vi "chem_shift.vi"() -> ()   [LabVIEW 2014]
uses:
  <vilib>/Analysis/6fits.llb/Curve Fitting Criteria.ctl
  <vilib>/Utility/file.llb/Write To Spreadsheet File (I64).vi
  <vilib>/Utility/file.llb/Write To Spreadsheet File (DBL).vi
  <vilib>/Analysis/NI_AALPro.lvlib
panel:
  in  "semester":string(combo)="ws17"
  out "ppm4":dbl=nan format="%.1f"
  out "peak4 [Hz]":dbl=nan format="%.1f"
  in  "W4-high [Hz]":i32
  in  "W4-low [Hz]":i32
  out "ppm3":dbl=nan format="%.1f"
  out "peak3 [Hz]":dbl=nan format="%.1f"
  in  "W3-high [Hz]":i32
  in  "W3-low [Hz]":i32
  out "ppm2":dbl=nan format="%.1f"
  out "peak2 [Hz]":dbl=nan format="%.1f"
  in  "W2-high [Hz]":i32
  in  "W2-low [Hz]":i32
  out "XY Graph":cluster{"Y":dbl[], "Y":dbl[]}[](graph)
  in  "meas":bool=TRUE
  out "Amplitude":cluster{"Y":dbl[], "Y":dbl[]}[](graph)
  out "Fourier transform":cluster{"Y":dbl[], "Y":dbl[]}[](graph)
  out "ppm1":dbl=nan format="%.1f"
  out "peak1 [Hz]":dbl=nan format="%.1f"
  out "offset":i32=4
  out "del freq":u32=2
  in  "W1-high [Hz]":i32
  in  "W1-low [Hz]":i32
  in  "fit:":bool=TRUE
  in  "folder":string
  in  "data file":string
  in  "scan freq [kHz]":u32=10
  in  "stop":bool=TRUE
  # "1)"
  # "2)"
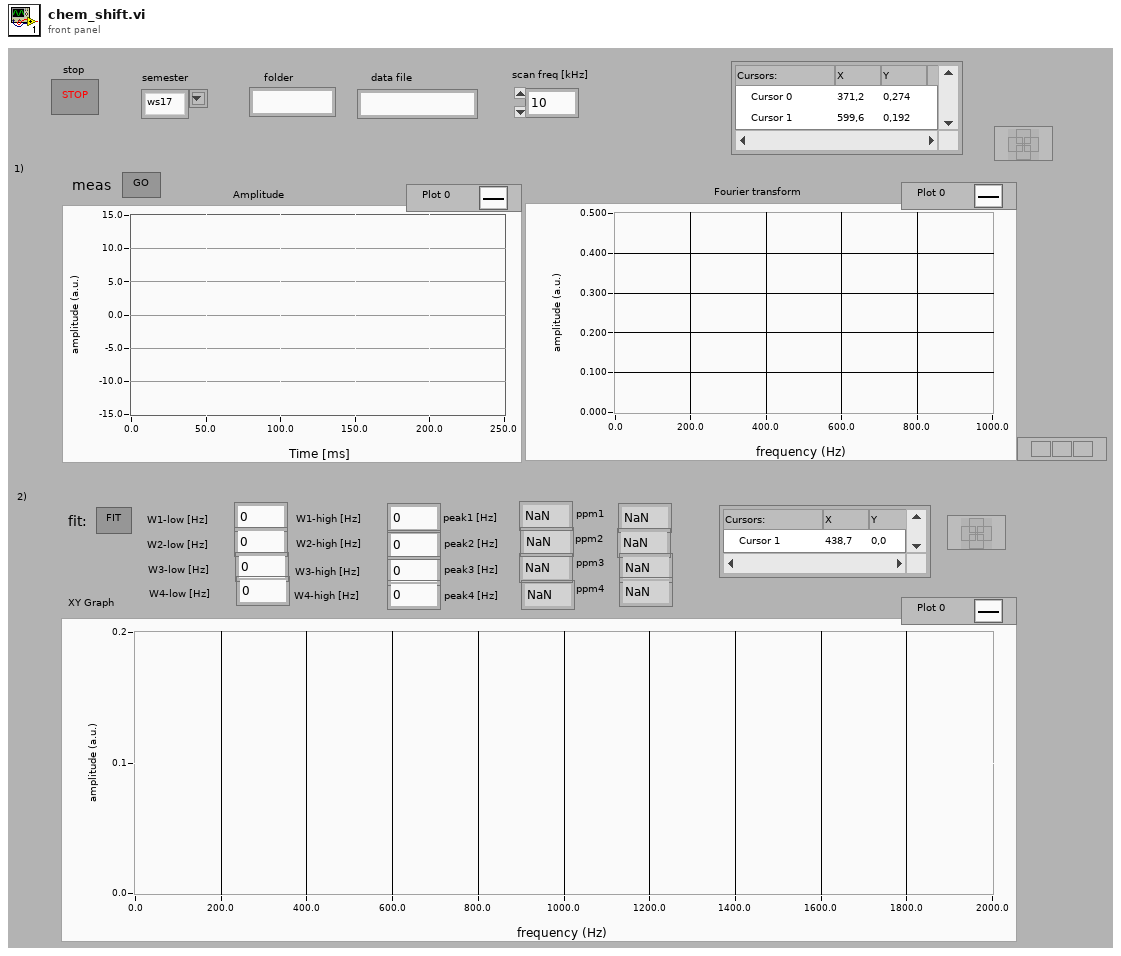
[diagram p1: front panel]
types:
  T1 = enum16{"open", "replace", "create", "open or create", "replace or create", "replace or create with confirmation"}
  T2 = typedef "NI_AALPro.lvlib/Curve Fitting Criteria.ctl" = u16
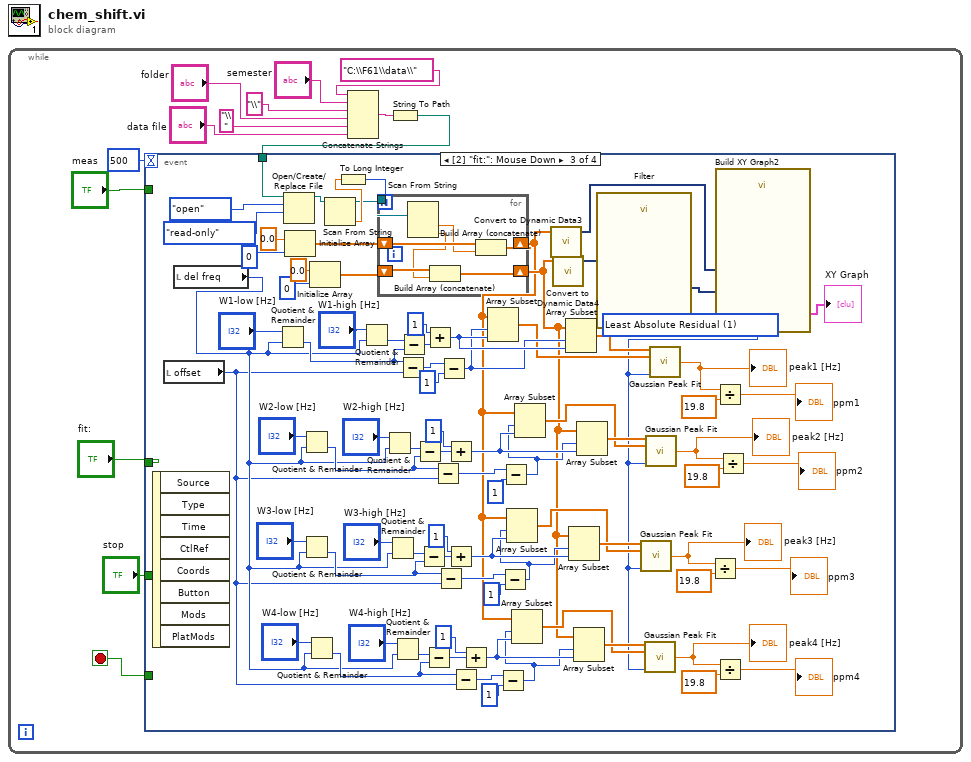
[diagram p0: block diagram]
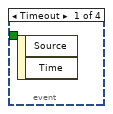
[diagram p2: hidden frame]
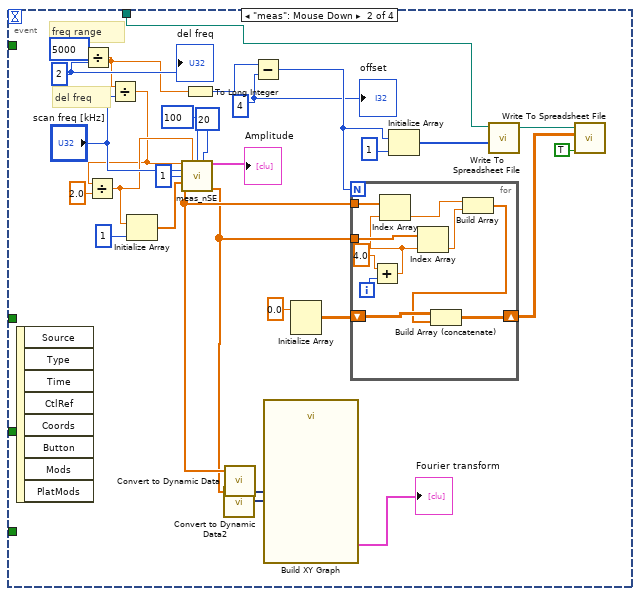
[diagram p3: hidden frame]
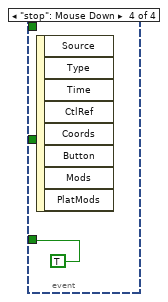
[diagram p4: hidden frame]
diagram:
  n1 = while {
    stop <- w11 stop-if-true
    n2 = Concatenate Strings("C:\\F61\\data\\", "semester", "\\" ("string"), "folder", "\\" ("string"), "data file") -> (w13:string)
    n3 = String To Path(string=w13) -> (path=w1:path)
    n4 = event shown="[2] \"fit:\": Mouse Down" {
      selector: _ -> [_ _ _ _]
      dyn-events: _ -> [_ _ _ _]
      timeout: 500 -> [_ _ _ _]
      tunnel: "meas" -> [_ _ _ _]
      tunnel: "fit:" -> [_ _ _ _]
      tunnel: "stop" -> [_ _ _ _]
      tunnel: [_ _ _ TRUE ("stop")] -> w11
      tunnel: w1 -> [_ w14 w53 _]
      event Timeout {
        n5 = event-data() -> ()  [unwired: 1 in, 2 out]
      }
      event "meas": Mouse Down {
        w17 = 4 ("y")
        w38 = u32 2 ("y")
        # "del freq"
        # "freq range"
        n6 = event-data() -> ()  [unwired: 1 in, 8 out]
        n7 = Divide(x=u32 5000, y=w38) -> (x/y=w19:dbl)
        n8 = Divide(x=w19, y="scan freq [kHz]") -> (x/y=w21:dbl)
        n9 = Divide(x=w21, y=2.0) -> (x/y=w35:dbl)
        n10 = Initialize Array(w35, 1 ("dimension size")) -> (w40:dbl[])
        n11 = call "meas_nSE.vi"("meas. time [ms]"=w21, "del T (+-) ][ms]"=w35, "gainfac"=u32 100, "time out [s]"=u32 20, "scan freq [kHz]"="scan freq [kHz]", "nr of SE"=u32 1, "SE-times"=w40) -> ("Amplitude"=→"Amplitude":cluster{"Y":dbl[], "Y":dbl[]}[], "xval"=w30:dbl[], "yval"=w29:dbl[])  [unwired: 3 in, 3 out]
        n12 = To Long Integer(number=w19) -> (32bit integer=w20:i32)
        n13 = call "Convert to Dynamic Data2"("Array"=w29) -> ("Dynamic Data Type"=w32:dynamicdata)  [unwired: 3 in]
        n14 = call "Convert to Dynamic Data"("Array"=w30) -> ("Dynamic Data Type"=w33:dynamicdata)  [unwired: 3 in]
        n15 = Subtract(x=w20, y=w17) -> (x-y=w18:i32)
        n16 = call "Build XY Graph"("Y Input"=w32, "X Input"=w33) -> ("XY Graph"=→"Fourier transform":cluster{"X":dbl[], "Y":dbl[]}[])  [unwired: 8 in, 1 out]
        n17 = Initialize Array(0.0 ("element")) -> (w27:dbl[][])  [unwired: 2 in]
        n18 = for {
          N: w18 -> [_]
          tunnel: w30 -> [w52]
          tunnel: w29 -> [w51]
          shift-right: [w44] -> w23
          shift-left: w27 -> [w45]
          i -> [w48]
          n19 = Add(x=4.0, y=w48) -> (x+y=w49:dbl)
          n20 = Index Array(array=w52, index=w49) -> (element=w47:dbl)
          n21 = Index Array(array=w51, index=w49) -> (element=w46:dbl)
          n22 = Build Array(w47, w46) -> (w43:dbl[])
          n23 = Build Array (concatenate)(w45, w43) -> (w44:dbl[][])
        }
        n24 = Initialize Array(w18, 1 ("dimension size")) -> (w25:i32[])
        n25 = call-poly <vilib>:"Write To Spreadsheet File.vi"("1D data"=w25, "file path (dialog if empty)"=w14) -> ("new file path (Not A Path if cancelled)"=w24:path)  [unwired: 6 in]
        n26 = call-poly <vilib>:"Write To Spreadsheet File.vi"("append to file? (new file:F)"=TRUE, "2D data"=w23, "file path (dialog if empty)"=w24) -> ()  [unwired: 5 in, 1 out]
        "del freq" <- w38
        "offset" <- w17
      }
      event "fit:": Mouse Down {
        w55 = T2 1 items=["Least Square", "Least Absolute Residual", "Bisquare"] ("method")
        n27 = event-data() -> ()  [unwired: 1 in, 8 out]
        n28 = local read "offset"() -> (w57:i32)
        n29 = local read "del freq"() -> (w58:u32)
        n30 = Quotient & Remainder(x="W1-low [Hz]", y=w58) -> (floor(x/y)=w117:u32)  [unwired: 1 out]
        n31 = Open/Create/Replace File(file path (use dialog)=w53, operation (0:open)=T1."open", access (0:read/write)=enum16{"read/write", "read-only", "write-only"}."read-only") -> (refnum out=w132:refnum<file>)  [unwired: 3 in, 2 out]
        n32 = Initialize Array(0.0 ("element"), 0 ("dimension size")) -> (w125:dbl[])
        n33 = Quotient & Remainder(x="W2-low [Hz]", y=w58) -> (floor(x/y)=w98:u32)  [unwired: 1 out]
        n34 = Quotient & Remainder(x="W3-low [Hz]", y=w58) -> (floor(x/y)=w83:u32)  [unwired: 1 out]
        n35 = Quotient & Remainder(x="W4-low [Hz]", y=w58) -> (floor(x/y)=w68:u32)  [unwired: 1 out]
        n36 = Initialize Array(0.0 ("element"), 0 ("dimension size")) -> (w124:dbl[])
        n37 = Scan From String(w132) -> (w123:refnum<file>, output 1=w130:dbl)  [unwired: 3 in, 1 out]
        n38 = To Long Integer(number=w130) -> (32bit integer=w131:i32)
        n39 = Quotient & Remainder(x="W1-high [Hz]", y=w58) -> (floor(x/y)=w116:u32)  [unwired: 1 out]
        n40 = for {
          N: w131 -> [_]
          shift-right: [w138] -> w56
          shift-left: w124 -> [w139]
          shift-right: [w140] -> w54
          shift-left: w125 -> [w141]
          tunnel: w123 -> [w137]
          n41 = Scan From String(w137) -> (output 1=w136:dbl, output 2=w135:dbl)  [unwired: 4 in, 2 out]
          n42 = Build Array (concatenate)(w139, w135) -> (w138:dbl[])
          n43 = Build Array (concatenate)(w141, w136) -> (w140:dbl[])
        }
        n44 = Quotient & Remainder(x="W2-high [Hz]", y=w58) -> (floor(x/y)=w99:u32)  [unwired: 1 out]
        n45 = Quotient & Remainder(x="W3-high [Hz]", y=w58) -> (floor(x/y)=w84:u32)  [unwired: 1 out]
        n46 = Quotient & Remainder(x="W4-high [Hz]", y=w58) -> (floor(x/y)=w69:u32)  [unwired: 1 out]
        n47 = Subtract(x=w117, y=w57) -> (x-y=w115:u32)
        n48 = Subtract(x=w116, y=w117) -> (x-y=w120:u32)
        n49 = Subtract(x=w99, y=w98) -> (x-y=w101:u32)
        n50 = Subtract(x=w84, y=w83) -> (x-y=w86:u32)
        n51 = Subtract(x=w69, y=w68) -> (x-y=w71:u32)
        n52 = Add(x=u32 1, y=w120) -> (x+y=w118:u32)
        n53 = Subtract(x=w98, y=w57) -> (x-y=w97:u32)
        n54 = Subtract(x=w83, y=w57) -> (x-y=w82:u32)
        n55 = Subtract(x=w115, y=u32 1) -> (x-y=w113:u32)
        n56 = Add(x=u32 1, y=w101) -> (x+y=w95:u32)
        n57 = Add(x=u32 1, y=w86) -> (x+y=w80:u32)
        n58 = Subtract(x=w68, y=w57) -> (x-y=w67:u32)
        n59 = Add(x=u32 1, y=w71) -> (x+y=w65:u32)
        n60 = Array Subset(array=w54, index=w113, length=w118) -> (w111:dbl[])
        n61 = Subtract(x=w67, y=u32 1) -> (x-y=w64:u32)
        n62 = Subtract(x=w82, y=u32 1) -> (x-y=w79:u32)
        n63 = Subtract(x=w97, y=u32 1) -> (x-y=w94:u32)
        n64 = Array Subset(array=w54, index=w79, length=w80) -> (w77:dbl[])
        n65 = Array Subset(array=w54, index=w64, length=w65) -> (w62:dbl[])
        n66 = Array Subset(array=w54, index=w94, length=w95) -> (w92:dbl[])
        n67 = call "Convert to Dynamic Data3"("Array"=w54) -> ("Dynamic Data Type"=w104:dynamicdata)  [unwired: 3 in]
        n68 = call "Convert to Dynamic Data4"("Array"=w56) -> ("Dynamic Data Type"=w106:dynamicdata)  [unwired: 3 in]
        n69 = Array Subset(array=w56, index=w113, length=w118) -> (w112:dbl[])
        n70 = Array Subset(array=w56, index=w79, length=w80) -> (w78:dbl[])
        n71 = Array Subset(array=w56, index=w64, length=w65) -> (w63:dbl[])
        n72 = Array Subset(array=w56, index=w94, length=w95) -> (w93:dbl[])
        n73 = call "Filter"("Signal"=w106) -> ("Filtered Signal"=w105:dynamicdata)  [unwired: 9 in, 1 out]
        n74 = call <vilib>:"Gaussian Peak Fit.vi"("Y"=w78, "X"=w77, "method"=w55) -> ("center"=w74:dbl)  [unwired: 6 in, 6 out]
        "peak3 [Hz]" <- w74
        n75 = call <vilib>:"Gaussian Peak Fit.vi"("Y"=w63, "X"=w62, "method"=w55) -> ("center"=w59:dbl)  [unwired: 6 in, 6 out]
        "peak4 [Hz]" <- w59
        n76 = call <vilib>:"Gaussian Peak Fit.vi"("Y"=w93, "X"=w92, "method"=w55) -> ("center"=w89:dbl)  [unwired: 6 in, 6 out]
        "peak2 [Hz]" <- w89
        n77 = call <vilib>:"Gaussian Peak Fit.vi"("Y"=w112, "X"=w111, "method"=w55) -> ("center"=w110:dbl)  [unwired: 6 in, 6 out]
        "peak1 [Hz]" <- w110
        n78 = Divide(x=w74, y=19.8) -> (x/y=→"ppm3":dbl)
        n79 = Divide(x=w110, y=19.8) -> (x/y=→"ppm1":dbl)
        n80 = Divide(x=w59, y=19.8) -> (x/y=→"ppm4":dbl)
        n81 = call "Build XY Graph2"("Y Input"=w105, "X Input"=w104) -> ("XY Graph"=→"XY Graph":cluster{"X":dbl[], "Y":dbl[]}[])  [unwired: 8 in, 1 out]
        n82 = Divide(x=w89, y=19.8) -> (x/y=→"ppm2":dbl)
      }
      event "stop": Mouse Down {
        n83 = event-data() -> ()  [unwired: 1 in, 8 out]
      }
    }
  }
